vi "pco.labview_Live_Example.vi"() -> ()   [LabVIEW 2019]
doc: "A short program to demonstrate the fundamentals of control and image acquision with the pco.camera series. The program records a sequence of images, with \"live\" updating, until the \"StopRecording\" button is pressed. Use ctrl-H for more help on the individual controls and indicators.\n\nCopyright 2004, 2010 The Cooke Corporation."
uses:
  pco.sdk/CameraAccess/CameraAccess.lvlib
  pco.sdk/ImageSensor/ImageSensor.lvlib
  pco.sdk/TimingControl/TimingControl.lvlib
  pco.recorder/Recorder.lvlib
  pco.sdk/RecordingControl/RecordingControl.lvlib
  pco.sdk/CameraDescription/CameraDescription.lvlib
  pco.sdk/GeneralCameraControl/GeneralCameraControl.lvlib
panel:
  out "Recorded Images":u32
  in  "TriggerMode":u16(ring) items=["auto sequence"=0, "software trigger"=1, "external exposure start & software trigger"=2, "external exposure control"=3, "external synchronized"=4, "fast external exposure control"=5, "external CDS control"=6, "slow external exposure control"=7, "external synchronized HDSDI"=258]
  in  "Quit":bool
  out "Image":u16[][](graph)
  out "Error":errorcluster {"code" format="%x"}
  in  "Stop Record":bool
  out "Recording On":bool
  in  "roiY1":u16=2 min=2 max=5120 step=1
  in  "roiX1":u16=2 min=2 max=896 step=1
  in  "roiY0":u16=1 min=1 max=5119 step=1
  in  "roiX0":u16=1 min=1 max=895 step=1
  out "Image Height":u16
  out "Image Width":u16
  in  "Image Index":u32 max=9
  in  "dwImgCount":u32=10 caption="Required Number of Images" max=2397
  in  "DelayTimeBase":u16(ring)=2 items=["nanoseconds", "microseconds", "milliseconds"]
  in  "ExposureTimeBase":u16(ring)=2 items=["nanoseconds", "microseconds", "milliseconds"]
  in  "Exposure":u32=10 min=1
  in  "Delay":u32
  in  "Rate":i32(ring) items=["Low", "High"]
  # "This example demonstrates the image acquisition with one camera in ring buffer mode together with a live display of the latest images during record. After record is stopped, the images can be addressed by index.\nNote that this example will not be fail save, i.e. doesnt react on errors, just handles them forward to the end\n\nUsage:\nSelect your required image count and the camera setup before you start the program.\nOnce started, the camera will be opened, the recorder will be created, initialized and images will be recorded and displayed automatically\nYou can stop the images by pressing stop record.\nAfter stopped, the image at the selected index will be read out\nTo finish the program click on quit application, this will force free and delete of the recorder and a close camera\nYou can change your required ROI after and also during the record."
  # "pco.labview"
  # "Camera Setup"
  # "Recording Control"
  # "Parameters for image readout"
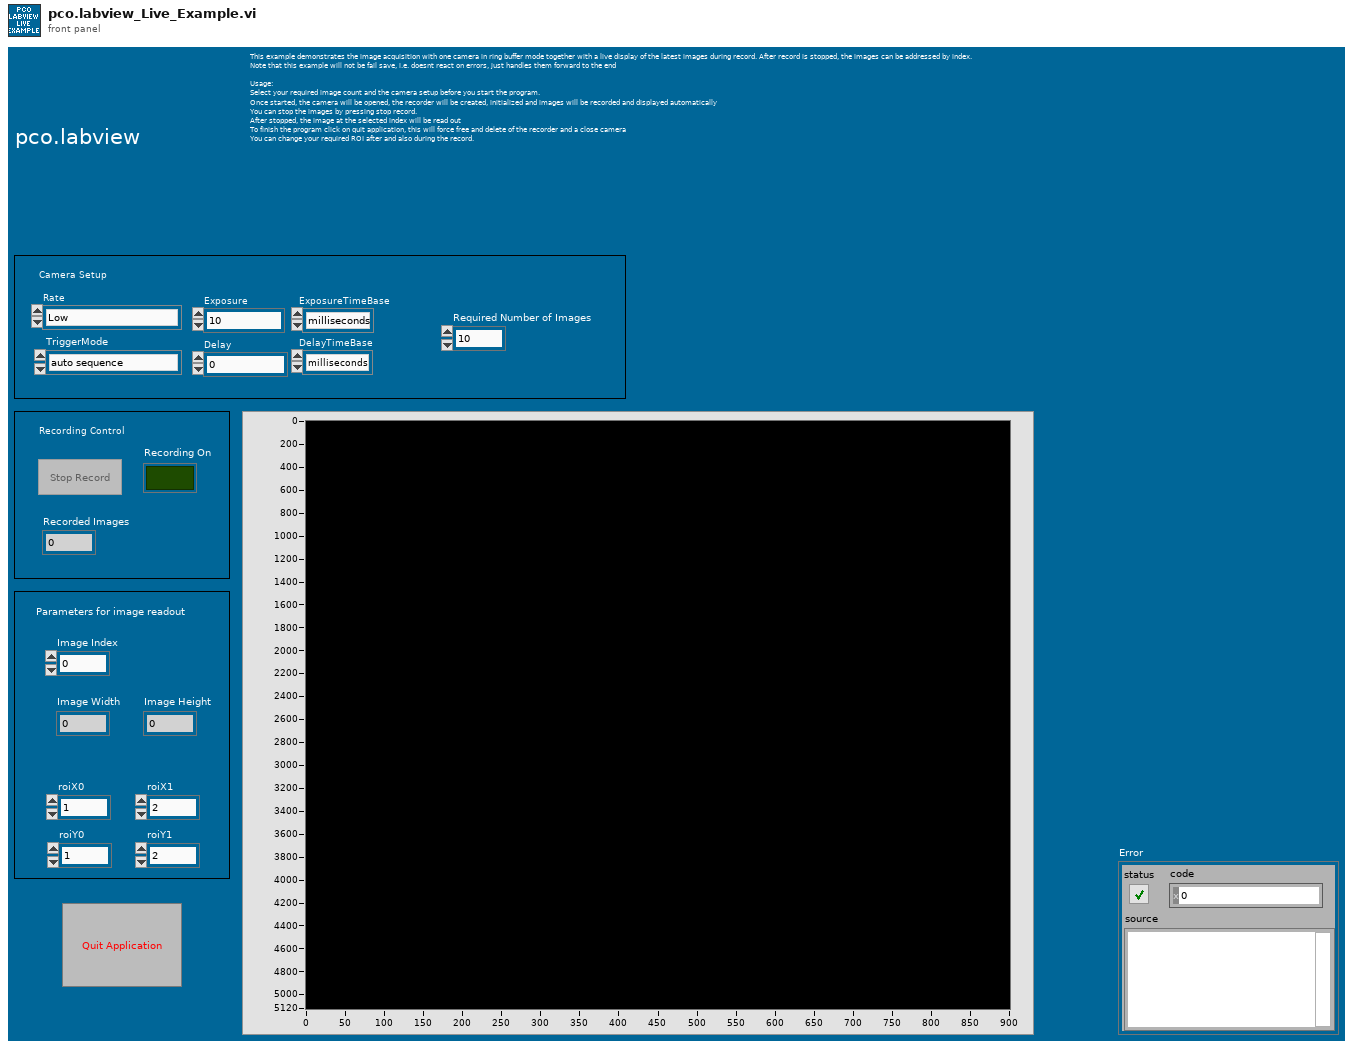
[diagram p1: front panel]
types:
  T1 = enum8{"Enabled", "Disabled", "Disabled and Grayed Out"}
  T2 = cluster{"wSensorTypeDESC":u16, "wSensorSubTypeDESC":u16, "wMaxHorzResStdDESC":u16, "wMaxVertResStdDESC":u16, "wMaxHorzResExtDESC":u16, "wMaxVertResExtDESC":u16, "wDynResDESC":u16, "wMaxBinHorzDESC":u16, "wBinHorzSteppingDESC":u16, "wMaxBinVertDESC":u16, "wBinVertSteppingDESC":u16, "wRoiHorStepsDESC":u16, "wRoiVertStepsDESC":u16, "wNumADCsDESC":u16, "wMinSizeHorzDESC":u16, "dwPixelRateDESC":u32[], "wConvFactDESC":u16[], "sCoolingSetpoints":i16[], "wSoftRoiHorStepsDESC":u16, "wSoftRoiVertStepsDESC":u16, "wIRDESC":u16, "wMinSizeVertDESC":u16, "dwMinDelayDESC":u32, "dwMaxDelayDESC":u32, "dwMinDelayStepDESC":u32, "dwMinExposureDESC":u32, "dwMaxExposureDESC":u32, "dwMinExposureStepDESC":u32, "dwMinDelayIRDESC":u32, "dwMaxDelayIRDESC":u32, "dwMinExposureIRDESC":u32, "dwMaxExposureIRDESC":u32, "wTimeTableDESC":u16, "wDoubleImageDESC":u16, "sMinCoolSetDESC":i16, "sMaxCoolSetDESC":i16, "sDefaultCoolSetDESC":i16, "wPowerDownModeDESC":u16, "wOffsetRegulationDESC":u16, "wColorPatternDESC":u16, "wPatternTypeDESC":u16, "wNumCoolingSetpoints":u16, "dwGeneralCapsDESC1":u32, "dwGeneralCapsDESC2":u32, "dwExtSyncFrequency":u32[], "dwGeneralCapsDESC3":u32, "dwGeneralCapsDESC4":u32}
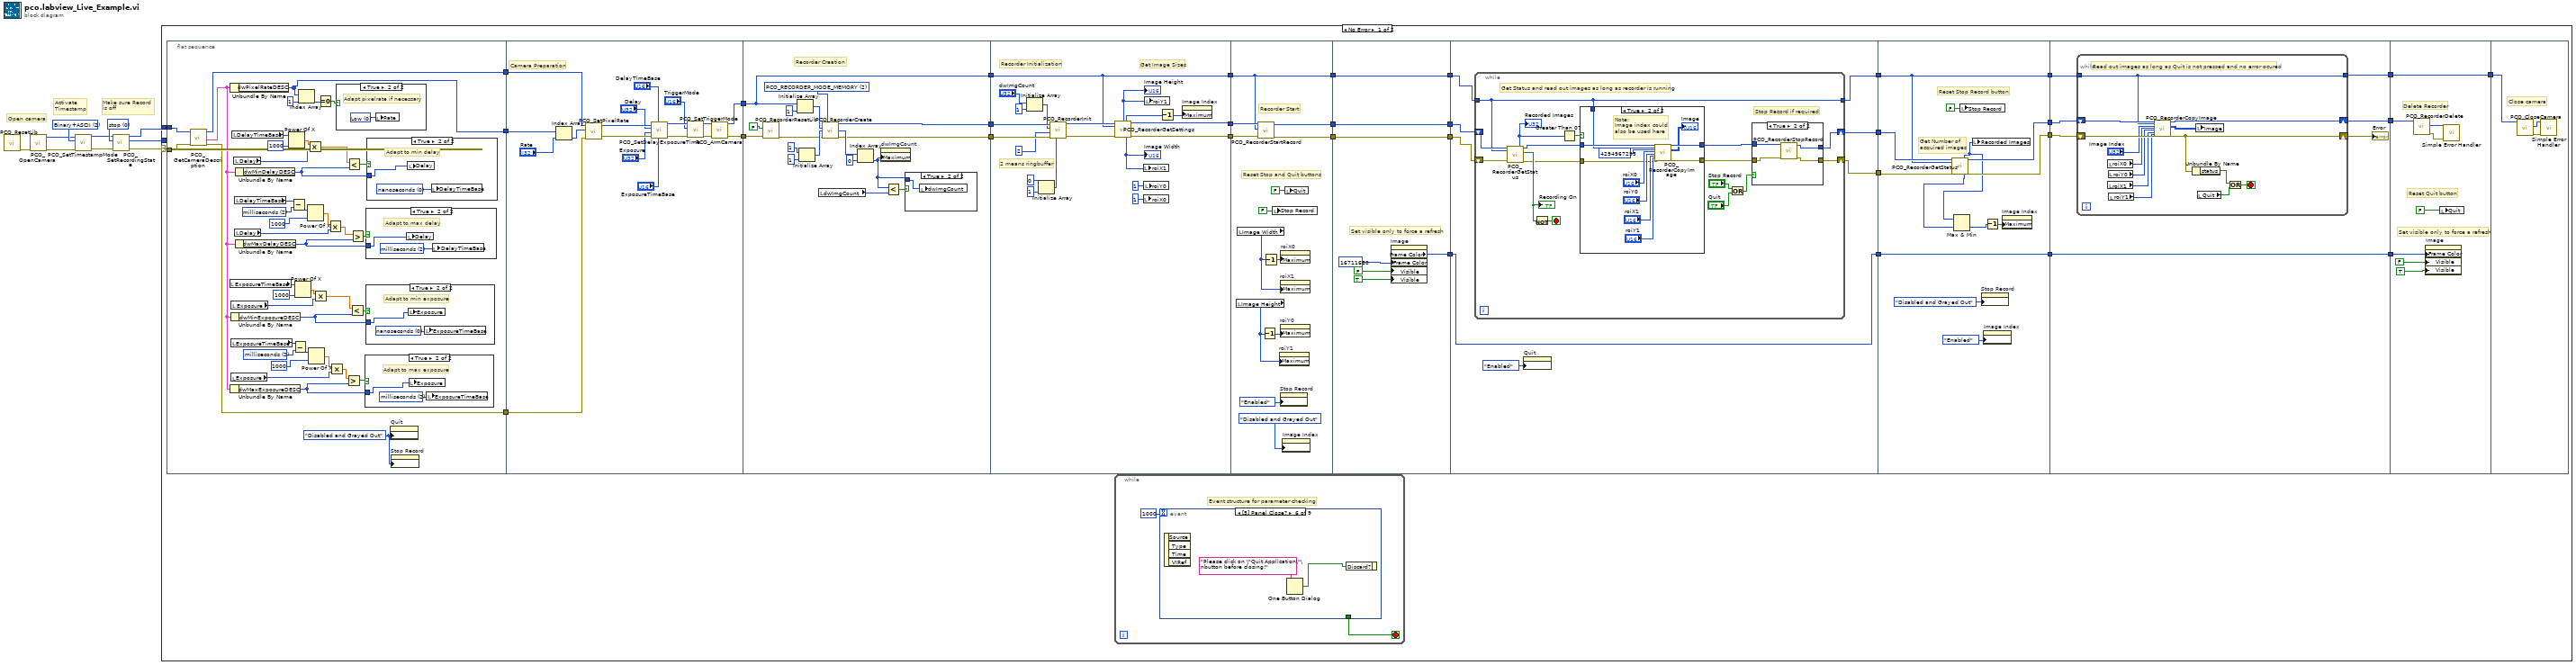
[diagram p0: block diagram]
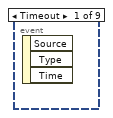
[diagram p2: hidden frame]
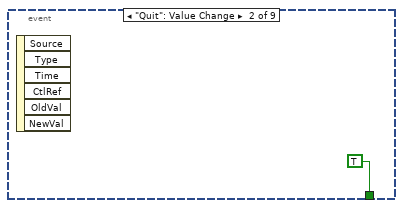
[diagram p3: hidden frame]
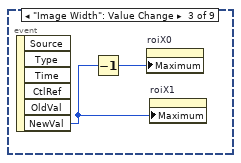
[diagram p4: hidden frame]
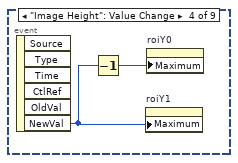
[diagram p5: hidden frame]
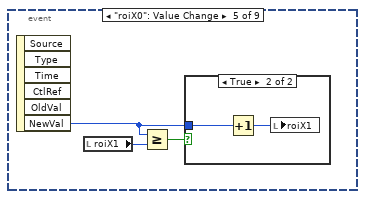
[diagram p6: hidden frame]
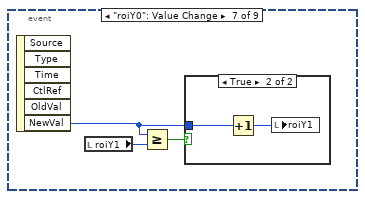
[diagram p8: hidden frame]
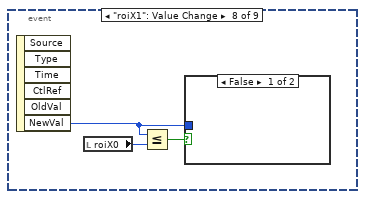
[diagram p10: hidden frame]
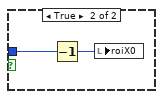
[diagram p11: hidden frame]
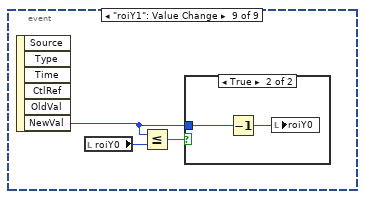
[diagram p12: hidden frame]
diagram:
  w5 = u16 2 items=["OFF", "Binary", "Binary+ASCII", "ASCII"] ("wTimeStampMode")
  w9 = u16 0 items=["stop", "run"] ("wRecState")
  # "Activate\nTimestamp"
  # "Make sure Record \nis off"
  # "Open camera"
  n1 = call "PCO_ResetLib.vi"() -> ("error out"=w10:errorcluster)  [unwired: 10 in, 1 out]
  n2 = call "PCO_OpenCamera.vi"("error in (no error)"=w10) -> ("error out"=w3:errorcluster, "ph out"=w4:u64)  [unwired: 8 in, 1 out]
  n3 = call "PCO_SetTimestampMode.vi"("error in (no error)"=w3, "wTimeStampMode"=w5, "ph"=w4) -> ("error out"=w2:errorcluster, "ph out"=w1:u64)  [unwired: 6 in, 1 out]
  n4 = call "PCO_SetRecordingState.vi"("error in (no error)"=w2, "wRecState"=w9, "ph"=w1) -> ("error out"=w7:errorcluster, "ErrorMessage"=w6:i32, "ph out"=w8:u64)  [unwired: 6 in]
  n5 = case shown="No Error" w7 {
    selector: w7 -> [w41 w288]
    tunnel: w8 -> [w42 _]
    tunnel: w6 -> [_ w287]
    frame No Error {
      n6 = flat-sequence {
        tunnel: w41 -> [w110]
        tunnel: w42 -> [w111]
        tunnel: [w106] -> w13
        tunnel: [w113] -> w12
        tunnel: [w112] -> w11
        tunnel: [w123] -> w40
        tunnel: [w124] -> w39
        tunnel: w13 -> [w129]
        tunnel: w12 -> [w128]
        tunnel: w11 -> [w127]
        tunnel: w40 -> [w156]
        tunnel: w39 -> [w145]
        tunnel: [w147] -> w38
        tunnel: [w146] -> w37
        tunnel: [w145] -> w34
        tunnel: w38 -> [w178]
        tunnel: w37 -> [w177]
        tunnel: [w168] -> w36
        tunnel: [w169] -> w35
        tunnel: w34 -> [w167]
        tunnel: [w167] -> w33
        tunnel: w36 -> [w189]
        tunnel: w35 -> [w188]
        tunnel: [w187] -> w23
        tunnel: [w186] -> w21
        tunnel: w33 -> [w185]
        tunnel: [w185] -> w19
        tunnel: w23 -> [w192]
        tunnel: [w192] -> w22
        tunnel: w21 -> [w193]
        tunnel: [w193] -> w20
        tunnel: w19 -> [w194]
        tunnel: [w194] -> w18
        tunnel: [w195] -> w17
        tunnel: w22 -> [w206]
        tunnel: w20 -> [w204]
        tunnel: w18 -> [w205]
        tunnel: [w203] -> w31
        tunnel: [w202] -> w29
        tunnel: [w201] -> w27
        tunnel: w17 -> [w199]
        tunnel: [w199] -> w16
        tunnel: [w249] -> w32
        tunnel: w31 -> [w250]
        tunnel: [w251] -> w30
        tunnel: w29 -> [w252]
        tunnel: [w248] -> w28
        tunnel: w27 -> [w248]
        tunnel: w16 -> [w253]
        tunnel: [w253] -> w14
        tunnel: w32 -> [w261]
        tunnel: w30 -> [w260]
        tunnel: w28 -> [w259]
        tunnel: [w257] -> w26
        tunnel: [w256] -> w25
        tunnel: [w255] -> w15
        tunnel: w14 -> [w255]
        tunnel: w26 -> [w282]
        tunnel: w25 -> [w279]
        tunnel: [w279] -> w24
        tunnel: w15 -> [w276]
        tunnel: w24 -> [w286]
        frame #0 {
          w77 = u16 2 items=["nanoseconds", "microseconds", "milliseconds"] ("DelayTimeBase")
          w91 = u16 2 items=["nanoseconds", "microseconds", "milliseconds"] ("DelayTimeBase")
          w100 = T1."Disabled and Grayed Out" ("Disabled")
          n7 = call "PCO_GetCameraDescription.vi"("error in (no error)"=w110, "ph"=w111) -> ("error out"=w113:errorcluster, "strDescription"=w101:T2, "ph out"=w112:u64)  [unwired: 6 in, 1 out]
          n8 = local read "ExposureTimeBase"() -> (w85:u16)
          n9 = Unbundle By Name(w101) -> ("dwPixelRateDESC"=w106:u32[])
          n10 = Unbundle By Name(w101) -> ("dwMaxExposureDESC"=w103:u32)
          n11 = Unbundle By Name(w101) -> ("dwMinExposureDESC"=w102:u32)
          n12 = local read "ExposureTimeBase"() -> (w76:u16)
          n13 = local read "Exposure"() -> (w74:u32)
          n14 = local read "Exposure"() -> (w82:u32)
          n15 = local read "DelayTimeBase"() -> (w96:u16)
          n16 = local read "Delay"() -> (w95:u32)
          n17 = local read "DelayTimeBase"() -> (w92:u16)
          n18 = local read "Delay"() -> (w88:u32)
          n19 = Unbundle By Name(w101) -> ("dwMinDelayDESC"=w105:u32)
          n20 = Unbundle By Name(w101) -> ("dwMaxDelayDESC"=w104:u32)
          n21 = Power Of X(1:u32 1000 ("Delay"), 2:w96) -> (0:w99:dbl)
          n22 = Subtract(x=w92, y=w91) -> (x-y=w93:i32)
          n23 = Subtract(x=w76, y=w77) -> (x-y=w75:i32)
          n24 = Power Of X(1:u32 1000 ("Delay"), 2:w85) -> (0:w83:dbl)
          n25 = Index Array(array=w106, index=1) -> (element=w108:u32)
          n26 = Multiply(x=w99, y=w95) -> (x*y=w94:dbl)
          n27 = Power Of X(1:u32 1000 ("Delay"), 2:w93) -> (0:w89:dbl)
          n28 = Power Of X(1:u32 1000 ("Delay"), 2:w75) -> (0:w79:dbl)
          n29 = Multiply(x=w83, y=w82) -> (x*y=w81:dbl)
          n30 = Equal To 0?(x=w108) -> (x = 0?=w107:bool)
          n31 = Multiply(x=w89, y=w88) -> (x*y=w87:dbl)
          n32 = Multiply(x=w79, y=w74) -> (x*y=w73:dbl)
          n33 = case shown="True" w107 {
            frame False {
            }
            frame True {
              w122 = 0 items=["Low", "High"] ("Rate")
              # "Adapt pixelrate if necessary"
              n34 = local write "Rate"(w122) -> ()
            }
          }
          n35 = Greater?(x=w73, y=w103) -> (0:w80:bool)
          n36 = Less?(x=w94, y=w105) -> (x < y?=w98:bool)
          n37 = Less?(x=w81, y=w102) -> (x < y?=w86:bool)
          n38 = Greater?(x=w87, y=w104) -> (0:w72:bool)
          n39 = case shown="True" w80 {
            tunnel: w103 -> [_ w115]
            frame False {
            }
            frame True {
              w114 = u16 2 items=["nanoseconds", "microseconds", "milliseconds"] ("DelayTimeBase")
              # "Adapt to max exposure"
              n40 = local write "Exposure"(w115) -> ()
              n41 = local write "ExposureTimeBase"(w114) -> ()
            }
          }
          n42 = case shown="True" w72 {
            tunnel: w104 -> [_ w119]
            frame False {
            }
            frame True {
              w118 = u16 2 items=["nanoseconds", "microseconds", "milliseconds"] ("DelayTimeBase")
              # "Adapt to max delay"
              n43 = local write "Delay"(w119) -> ()
              n44 = local write "DelayTimeBase"(w118) -> ()
            }
          }
          n45 = case shown="True" w86 {
            tunnel: w102 -> [_ w117]
            frame False {
            }
            frame True {
              w116 = u16 0 items=["nanoseconds", "microseconds", "milliseconds"] ("DelayTimeBase")
              # "Adapt to min exposure"
              n46 = local write "Exposure"(w117) -> ()
              n47 = local write "ExposureTimeBase"(w116) -> ()
            }
          }
          n48 = case shown="True" w98 {
            tunnel: w105 -> [_ w121]
            frame False {
            }
            frame True {
              w120 = u16 0 items=["nanoseconds", "microseconds", "milliseconds"] ("DelayTimeBase")
              # "Adapt to min delay"
              n49 = local write "Delay"(w121) -> ()
              n50 = local write "DelayTimeBase"(w120) -> ()
            }
          }
          n51 = property on="Quit" class="Bool (strict)"("DisabledEnum"=w100) -> ()  [unwired: 2 in, 2 out]
          n52 = property on="Stop Record" class="Bool (strict)"("DisabledEnum"=w100) -> ()  [unwired: 2 in, 2 out]
        }
        frame #1 {
          # "Camera Preparation"
          n53 = Index Array(array=w129, index="Rate") -> (element=w139:u32)
          n54 = call "PCO_SetPixelRate.vi"("error in (no error)"=w128, "dwPixelRate"=w139, "ph"=w127) -> ("error out"=w137:errorcluster, "ph out"=w138:u64)  [unwired: 6 in, 1 out]
          n55 = call "PCO_SetDelayExposureTime.vi"("wTimeBaseExposure"="ExposureTimeBase", "wTimeBaseDelay"="DelayTimeBase", "error in (no error)"=w137, "dwExposure"="Exposure", "dwDelay"="Delay", "ph"=w138) -> ("error out"=w131:errorcluster, "ph out"=w132:u64)  [unwired: 3 in, 1 out]
          n56 = call "PCO_SetTriggerMode.vi"("error in (no error)"=w131, "wTriggerMode"="TriggerMode", "ph"=w132) -> ("error out"=w125:errorcluster, "ph out"=w126:u64)  [unwired: 6 in, 1 out]
          n57 = call "PCO_ArmCamera.vi"("error in (no error)"=w125, "ph"=w126) -> ("error out"=w123:errorcluster, "ph out"=w124:u64)  [unwired: 7 in, 1 out]
        }
        frame #2 {
          w141 = u16 2 items=["PCO_RECORDER_MODE_FILE"=1, "PCO_RECORDER_MODE_MEMORY"=2, "PCO_RECORDER_MODE_CAMRAM"=3] ("dwRecMode")
          # "Recorder Creation"
          n58 = call "PCO_RecorderResetLib.vi"("error in (no error)"=w156, "bSilent"=FALSE) -> ("error out"=w148:errorcluster)  [unwired: 8 in, 1 out]
          n59 = Initialize Array(w145, 1 ("dimension size")) -> (w154:u64[])
          n60 = Initialize Array(u32 1 ("dimension size"), 1 ("dimension size")) -> (w151:u32[])
          n61 = local read "dwImgCount"() -> (w142:u32)
          n62 = call "PCO_RecorderCreate.vi"("wRecMode"=w141, "phCamArr"=w154, "dwImgDistributionArr"=w151, "error in (no error)"=w148) -> ("phRec out"=w146:u64, "dwMaxImgCountArr"=w150:u32[], "error out"=w147:errorcluster)  [unwired: 8 in, 1 out]
          n63 = Index Array(array=w150, index=0) -> (element=w143:u32)
          n64 = property on="dwImgCount" class="DigNum (strict)"("Maximum"=w143) -> ()  [unwired: 2 in, 2 out]
          n65 = Less?(x=w143, y=w142) -> (x < y?=w144:bool)
          n66 = case shown="True" w144 {
            tunnel: w143 -> [_ w158]
            frame False {
            }
            frame True {
              n67 = local write "dwImgCount"(w158) -> ()
            }
          }
        }
        frame #3 {
          # "2 means ringbuffer"
          # "Get Image Sizes"
          # "Recorder Initialization"
          n68 = Initialize Array("dwImgCount", 1 ("dimension size")) -> (w174:u32[])
          n69 = Initialize Array(u16 0 ("element"), 1 ("dimension size")) -> (w159:u16[])
          n70 = call "PCO_RecorderInit.vi"("wRamSegmentArr"=w159, "error in (no error)"=w178, "wType"=u16 2, "dwImgCountArr"=w174, "phRec"=w177) -> ("error out"=w173:errorcluster, "phRec out"=w172:u64)  [unwired: 4 in, 1 out]
          n71 = call "PCO_RecorderGetSettings.vi"("phRec"=w172, "phCam"=w167, "error in (no error)"=w173) -> ("wHeight"=w166:u16, "dwReqImgCount"=w163:u32, "phRec out"=w168:u64, "wWidth"=w165:u16, "error out"=w169:errorcluster)  [unwired: 4 in, 4 out]
          "Image Height" <- w166
          "Image Width" <- w165
          n72 = local write "roiX1"(w165) -> ()
          n73 = local write "roiX0"(u16 1 ("roiY0")) -> ()
          n74 = local write "roiY0"(u16 1 ("roiY0")) -> ()
          n75 = local write "roiY1"(w166) -> ()
          n76 = Decrement(x=w163) -> (x-1=w164:u32)
          n77 = property on="Image Index" class="DigNum (strict)"("Maximum"=w164) -> ()  [unwired: 2 in, 2 out]
        }
        frame #4 {
          # "Reset Stop and Quit buttons"
          # "Recorder Start"
          n78 = local read "Image Height"() -> (w182:u16)
          n79 = local read "Image Width"() -> (w181:u16)
          n80 = call "PCO_RecorderStartRecord.vi"("error in (no error)"=w188, "phCam"=w185, "phRec"=w189) -> ("error out"=w187:errorcluster, "phRec out"=w186:u64)  [unwired: 6 in, 1 out]
          n81 = Decrement(x=w182) -> (x-1=w183:u16)
          n82 = Decrement(x=w181) -> (x-1=w184:u16)
          n83 = local write "Stop Record"(FALSE ("Stop Record")) -> ()
          n84 = property on="roiY1" class="DigNum (strict)"("Maximum"=w182) -> ()  [unwired: 2 in, 2 out]
          n85 = property on="roiX1" class="DigNum (strict)"("Maximum"=w181) -> ()  [unwired: 2 in, 2 out]
          n86 = property on="roiY0" class="DigNum (strict)"("Maximum"=w183) -> ()  [unwired: 2 in, 2 out]
          n87 = property on="Stop Record" class="Bool (strict)"("DisabledEnum"=T1."Enabled" ("Disabled")) -> ()  [unwired: 2 in, 2 out]
          n88 = property on="roiX0" class="DigNum (strict)"("Maximum"=w184) -> ()  [unwired: 2 in, 2 out]
          n89 = property on="Image Index" class="DigNum (strict)"("DisabledEnum"=T1."Disabled and Grayed Out" ("Disabled")) -> ()  [unwired: 2 in, 2 out]
          n90 = local write "Quit"(FALSE ("Stop")) -> ()
        }
        frame #5 {
          # "Set visible only to force a refresh"
          n91 = property on="Image" class="IntGraph (strict)"("Frame Color"=u32 16711680, "Visible"=FALSE, "Visible"=TRUE) -> ("Frame Color"=w195:u32)  [unwired: 2 in, 2 out]
        }
        frame #6 {
          n92 = while {
            tunnel: w205 -> [w211]
            shift-right: [w212] -> w202
            shift-left: w206 -> [w222]
            shift-right: [w213] -> w203
            shift-left: w204 -> [w218]
            tunnel: [w211] -> w201
            stop <- w217 stop-if-true
            # "Stop Record if required"
            # "Get Status and read out images as long as recorder is running"
            n93 = call "PCO_RecorderGetStatus.vi"("phRec"=w218, "phCam"=w211, "error in (no error)"=w222) -> ("dwProcImgCount"=w207:u32, "phRec out"=w220:u64, "bIsRunning"=w221:bool, "error out"=w219:errorcluster)  [unwired: 5 in, 8 out]
            "Recording On" <- w221
            "Recorded Images" <- w207
            n94 = Not(x=w221) -> (.not. x?=w217:bool)
            n95 = Greater Than 0?(x=w207) -> (x > 0?=w208:bool)
            n96 = case shown="True" w208 {
              tunnel: w220 -> [w224 w235]
              tunnel: w219 -> [w223 w229]
              tunnel: [w224 w228] -> w216
              tunnel: [w223 w227] -> w215
              tunnel: w211 -> [_ w226]
              frame False {
              }
              frame True {
                # "Note: \nImage index could \nalso be used here"
                n97 = call "PCO_RecorderCopyImage.vi"("phRec"=w235, "phCam"=w226, "dwImgIdx"=u32 4294967295, "wRoiX0"="roiX0", "wRoiY0"="roiY0", "wRoiX1"="roiX1", "wRoiY1"="roiY1", "error in (no error)"=w229) -> ("phRec out"=w228:u64, "wImgBuf"=→"Image":u16[][], "error out"=w227:errorcluster)  [unwired: 13 in, 4 out]
              }
            }
            n98 = Or(x="Stop Record", y="Quit") -> (x .or. y?=w214:bool)
            n99 = case shown="True" w214 {
              tunnel: w216 -> [w237 w241]
              tunnel: w215 -> [w236 w240]
              tunnel: [w237 w238] -> w213
              tunnel: [w236 w239] -> w212
              frame False {
              }
              frame True {
                n100 = call "PCO_RecorderStopRecord.vi"("error in (no error)"=w240, "phRec"=w241) -> ("error out"=w239:errorcluster, "phRec out"=w238:u64)  [unwired: 7 in, 1 out]
              }
            }
          }
          n101 = property on="Quit" class="Bool (strict)"("DisabledEnum"=T1."Enabled" ("Disabled")) -> ()  [unwired: 2 in, 2 out]
        }
        frame #7 {
          # "Get Number of \nacquired images"
          # "Reset Stop Record button"
          n102 = call "PCO_RecorderGetStatus.vi"("phRec"=w250, "phCam"=w248, "error in (no error)"=w252) -> ("dwProcImgCount"=w244:u32, "dwReqImgCount"=w245:u32, "phRec out"=w249:u64, "error out"=w251:errorcluster)  [unwired: 5 in, 8 out]
          n103 = Max & Min(x=w244, y=w245) -> (min(x,y)=w246:u32)  [unwired: 1 out]
          n104 = local write "Stop Record"(FALSE ("Stop Record")) -> ()
          n105 = local write "Recorded Images"(w244) -> ()
          n106 = property on="Stop Record" class="Bool (strict)"("DisabledEnum"=T1."Disabled and Grayed Out" ("Disabled")) -> ()  [unwired: 2 in, 2 out]
          n107 = property on="Image Index" class="DigNum (strict)"("DisabledEnum"=T1."Enabled" ("Disabled")) -> ()  [unwired: 2 in, 2 out]
          n108 = Decrement(x=w246) -> (x-1=w247:u32)
          n109 = property on="Image Index" class="DigNum (strict)"("Maximum"=w247) -> ()  [unwired: 2 in, 2 out]
        }
        frame #8 {
          n110 = while {
            shift-right: [w263] -> w258
            shift-left: w260 -> [w272]
            shift-right: [w264] -> w257
            shift-left: w261 -> [w271]
            tunnel: w259 -> [w262]
            tunnel: [w262] -> w256
            stop <- w273 stop-if-true
            # "Read out images as long as Quit is not pressed and no error ocured"
            n111 = local read "roiX0"() -> (w269:u16)
            n112 = local read "roiX1"() -> (w267:u16)
            n113 = local read "roiY0"() -> (w268:u16)
            n114 = local read "roiY1"() -> (w266:u16)
            n115 = call "PCO_RecorderCopyImage.vi"("phRec"=w271, "phCam"=w262, "dwImgIdx"="Image Index", "wRoiX0"=w269, "wRoiY0"=w268, "wRoiX1"=w267, "wRoiY1"=w266, "error in (no error)"=w272) -> ("phRec out"=w264:u64, "wImgBuf"=w265:u16[][], "error out"=w263:errorcluster)  [unwired: 13 in, 4 out]
            n116 = Unbundle By Name(w263) -> ("status"=w275:bool)
            n117 = local write "Image"(w265) -> ()
            n118 = local read "Quit"() -> (w274:bool)
            n119 = Or(x=w275, y=w274) -> (x .or. y?=w273:bool)
          }
          "Error" <- w258
        }
        frame #9 {
          # "Set visible only to force a refresh"
          # "Delete Recorder"
          # "Reset Quit button"
          n120 = call "PCO_RecorderDelete.vi"("phRec"=w282) -> ("error out"=w280:errorcluster, "ErrorMessage"=w281:i32)  [unwired: 9 in]
          n121 = property on="Image" class="IntGraph (strict)"("Frame Color"=w276, "Visible"=FALSE, "Visible"=TRUE) -> ()  [unwired: 2 in, 2 out]
          n122 = local write "Quit"(FALSE ("Stop Record")) -> ()
          n123 = call <vilib>:"Simple Error Handler.vi"("error code (no error:0)"=w281, "error in (no error)"=w280) -> ()  [unwired: 3 in, 5 out]
        }
        frame #10 {
          # "Close camera"
          n124 = call "PCO_CloseCamera.vi"("ph"=w286) -> ("error out"=w284:errorcluster, "ErrorMessage"=w285:i32)  [unwired: 9 in]
          n125 = call <vilib>:"Simple Error Handler.vi"("error code (no error:0)"=w285, "error in (no error)"=w284) -> ()  [unwired: 3 in, 5 out]
        }
      }
      n126 = while {
        stop <- w43 stop-if-true
        # "Event structure for parameter checking"
        n127 = event shown="[5] Panel Close?" {
          selector: _ -> [_ _ _ _ _ _ _ _ _]
          dyn-events: _ -> [_ _ _ _ _ _ _ _ _]
          timeout: 1000 -> [_ _ _ _ _ _ _ _ _]
          tunnel: [_ TRUE _ _ _ _ _ _ _] -> w43
          event Timeout {
            n128 = event-data() -> ()  [unwired: 1 in, 3 out]
          }
          event "Quit": Value Change {
            n129 = event-data() -> ()  [unwired: 1 in, 6 out]
          }
          event "Image Width": Value Change {
            n130 = event-data() -> ("NewVal"=w46:u16)  [unwired: 1 in, 5 out]
            n131 = Decrement(x=w46) -> (x-1=w47:u16)
            n132 = property on="roiX0" class="DigNum (strict)"("Maximum"=w47) -> ()  [unwired: 2 in, 2 out]
            n133 = property on="roiX1" class="DigNum (strict)"("Maximum"=w46) -> ()  [unwired: 2 in, 2 out]
          }
          event "Image Height": Value Change {
            n134 = event-data() -> ("NewVal"=w48:u16)  [unwired: 1 in, 5 out]
            n135 = Decrement(x=w48) -> (x-1=w49:u16)
            n136 = property on="roiY1" class="DigNum (strict)"("Maximum"=w48) -> ()  [unwired: 2 in, 2 out]
            n137 = property on="roiY0" class="DigNum (strict)"("Maximum"=w49) -> ()  [unwired: 2 in, 2 out]
          }
          event "roiX0": Value Change {
            n138 = event-data() -> ("NewVal"=w50:u16)  [unwired: 1 in, 5 out]
            n139 = local read "roiX1"() -> (w52:u16)
            n140 = Greater Or Equal?(x=w50, y=w52) -> (x >= y?=w51:bool)
            n141 = case shown="True" w51 {
              tunnel: w50 -> [_ w54]
              frame False {
              }
              frame True {
                n142 = Increment(x=w54) -> (x+1=w53:u16)
                n143 = local write "roiX1"(w53) -> ()
              }
            }
          }
          event Panel Close? {
            n144 = event-data() -> ()  [unwired: 1 in, 4 out]
            n145 = One Button Dialog(message="Please click on \"Quit Application\"\nbutton before closing!") -> (true=w55:bool)  [unwired: 1 in]
            n146 = event-data("Discard?"=w55) -> ()  [unwired: 1 in, 1 out]
          }
          event "roiY0": Value Change {
            n147 = event-data() -> ("NewVal"=w57:u16)  [unwired: 1 in, 5 out]
            n148 = local read "roiY1"() -> (w59:u16)
            n149 = Greater Or Equal?(x=w57, y=w59) -> (x >= y?=w58:bool)
            n150 = case shown="True" w58 {
              tunnel: w57 -> [_ w61]
              frame False {
              }
              frame True {
                n151 = Increment(x=w61) -> (x+1=w60:u16)
                n152 = local write "roiY1"(w60) -> ()
              }
            }
          }
          event "roiX1": Value Change {
            n153 = event-data() -> ("NewVal"=w62:u16)  [unwired: 1 in, 5 out]
            n154 = local read "roiX0"() -> (w64:u16)
            n155 = Less Or Equal?(x=w62, y=w64) -> (x <= y?=w63:bool)
            n156 = case shown="False" w63 {
              tunnel: w62 -> [_ w66]
              frame False {
              }
              frame True {
                n157 = Decrement(x=w66) -> (x-1=w65:u16)
                n158 = local write "roiX0"(w65) -> ()
              }
            }
          }
          event "roiY1": Value Change {
            n159 = event-data() -> ("NewVal"=w67:u16)  [unwired: 1 in, 5 out]
            n160 = local read "roiY0"() -> (w69:u16)
            n161 = Less Or Equal?(x=w67, y=w69) -> (x <= y?=w68:bool)
            n162 = case shown="True" w68 {
              tunnel: w67 -> [_ w71]
              frame False {
              }
              frame True {
                n163 = Decrement(x=w71) -> (x-1=w70:u16)
                n164 = local write "roiY0"(w70) -> ()
              }
            }
          }
        }
      }
    }
    frame Error {
      n165 = call <vilib>:"Simple Error Handler.vi"("error code (no error:0)"=w287, "error in (no error)"=w288) -> ()  [unwired: 3 in, 5 out]
    }
  }
